vi "DriveForward.vi"(0 "LeftEncoder":T13={"DevStatus"={"status"=FALSE, "code"=0, "source"=""}, "EncoderIndex"=enum."Invalid", "CounterIndex"=enum."Invalid", "DistancePerCount"=1.0, "Decoding Type"=enum."4x"}, 1 "RightEncoder":T13={"DevStatus"={"status"=FALSE, "code"=0, "source"=""}, "EncoderIndex"=enum."Invalid", "CounterIndex"=enum."Invalid", "DistancePerCount"=1.0, "Decoding Type"=enum."4x"}, 2 "Inches to Travel":dbl, 4 "Drive":T3={"DevStatus"={"status"=FALSE, "code"=0, "source"=""}, "Motors[]"=[], "Square Inputs"=FALSE, "Max Output"=1.0}, 5 "Max":dbl, 6 "Transmission":T1={"DevStatus"={"status"=FALSE, "code"=0, "source"=""}, "Pneumatics Control Module"=0, "Forward Solenoid Channel"=enum."Invalid", "Reverse Solenoid Channel"=enum."Invalid"}) -> ()   [LabVIEW 2014]
uses:
  <vilib>/Rock Robotics/WPI/Encoder/WPI_EncoderDevRef.ctl
  <vilib>/Rock Robotics/SystemInterfaces/Encoder/FPGA_EncoderIdx.ctl
  <vilib>/Rock Robotics/SystemInterfaces/Counter/FPGA_CounterCtrSystemIndex.ctl
  <vilib>/Rock Robotics/WPI/Encoder/WPI_EncoderType.ctl
  <vilib>/Rock Robotics/WPI/RobotDrive/WPI_RobotDriveDevRef.ctl
  <vilib>/Rock Robotics/WPI/MotorControl/WPI_MotorControlDeviceRef.ctl
  <vilib>/Rock Robotics/WPI/MotorControl/WPI_MotorControlType.ctl
  <vilib>/Rock Robotics/SystemInterfaces/Typedef/FPGA_TypedefDigitalModule.ctl
  <vilib>/Rock Robotics/SystemInterfaces/DIO/FPGA_DIOPWMChannel.ctl
  <vilib>/Rock Robotics/WPI/PWM/WPI_PWMDeadband.ctl
  <vilib>/Rock Robotics/WPI/CAN/Jaguar/SubVIs/WPI_CANJaguar_ControlMode.ctl
  <vilib>/Rock Robotics/WPI/CAN/TalonSRX/WPI_CANTalonSRX_APIControlMode.ctl
  <vilib>/Rock Robotics/WPI/PWM/WPI_PWMTransform_ConPane.ctl
  <vilib>/Rock Robotics/WPI/Solenoid/WPI_SolenoidDevRef.ctl
  <vilib>/Rock Robotics/WPI/Solenoid/WPI_SolenoidChannel.ctl
  <vilib>/addons/control/pid/pid.llb/PID (DBL).vi
  <vilib>/addons/control/pid/NI_PID_pid.lvlib
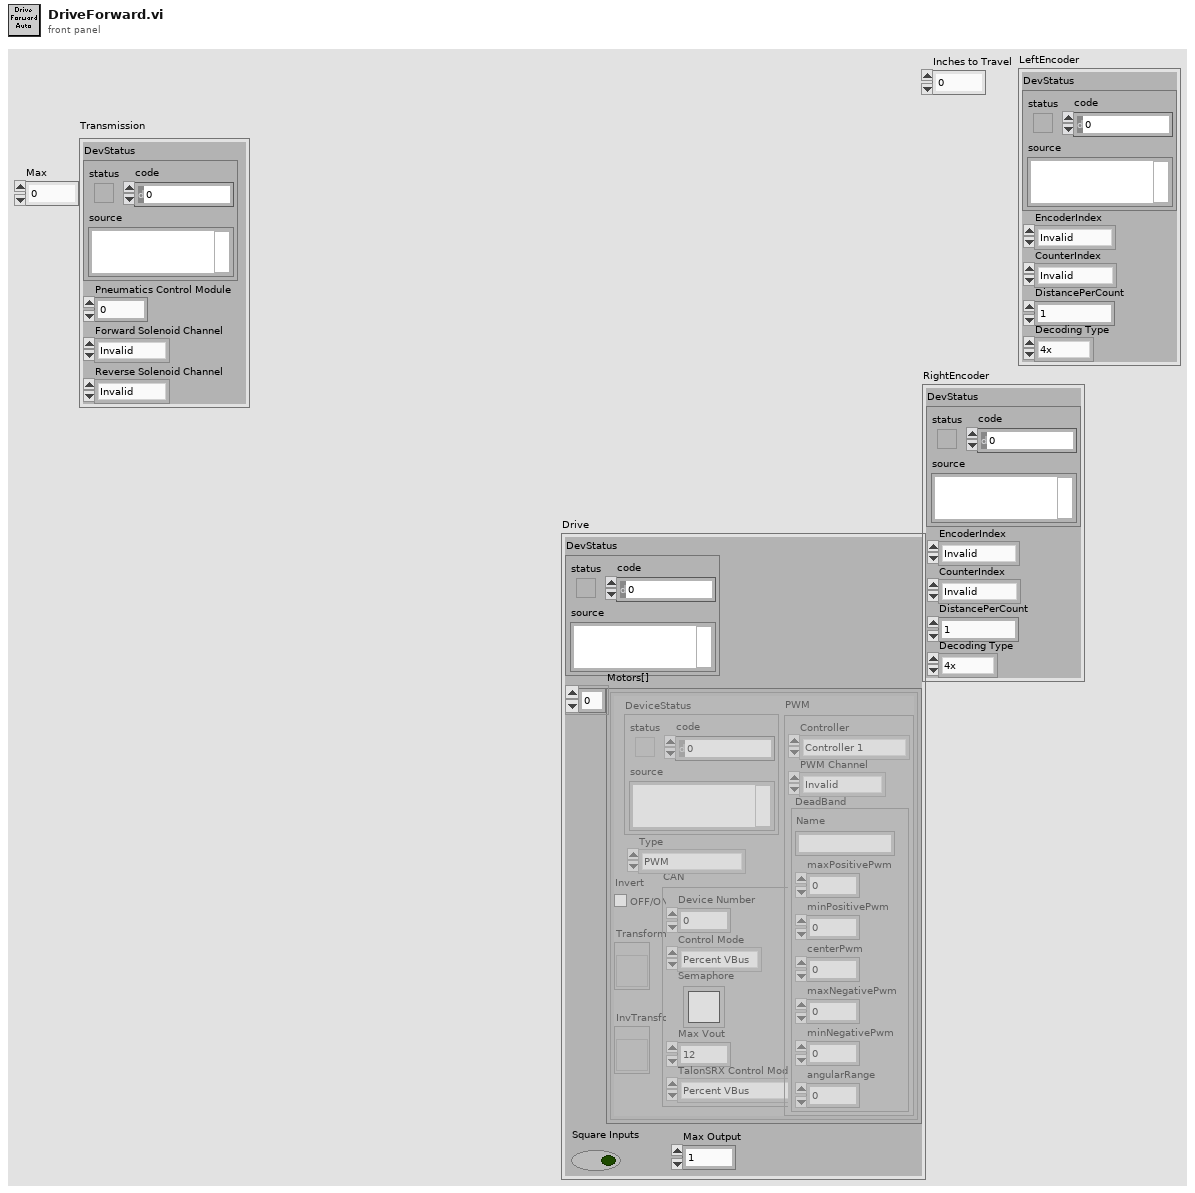
[diagram p1: front panel]
types:
  T1 = typedef "WPI_SolenoidDevRef.ctl" = cluster{"DevStatus":errorcluster, "Pneumatics Control Module":u8, "Forward Solenoid Channel":T2, "Reverse Solenoid Channel":T2}
  T2 = typedef "WPI_SolenoidChannel.ctl" = enum8{"Solenoid 0", "Solenoid 1", "Solenoid 2", "Solenoid 3", "Solenoid 4", "Solenoid 5", "Solenoid 6", "Solenoid 7", "Invalid"}
  T3 = typedef "WPI_RobotDriveDevRef.ctl" = cluster{"DevStatus":errorcluster, "Motors[]":T4[], "Square Inputs":bool, "Max Output":dbl}
  T4 = typedef "WPI_MotorControlDeviceRef.ctl" = cluster{"DeviceStatus":errorcluster, "Type":T5, "PWM":cluster{"Controller":T6, "PWM Channel":T7, "DeadBand":T8}, "CAN":cluster{"Device Number":u8, "Control Mode":T9, "Semaphore":T10, "Max Vout":dbl, "TalonSRX Control Mode":T11}, "Invert":bool, "TransformRef":T12, "InvTransformRef":T12}
  T5 = typedef "WPI_MotorControlType.ctl" = enum16{"PWM", "CAN", "CANTalonSRX"}
  T6 = typedef "FPGA_TypedefDigitalModule.ctl" = enum16{"Controller 1"}
  T7 = typedef "FPGA_DIOPWMChannel.ctl" = enum8{"PWM 0", "PWM 1", "PWM 2", "PWM 3", "PWM 4", "PWM 5", "PWM 6", "PWM 7", "PWM 8", "PWM 9", "PWM MXP 0", "PWM MXP 1", "PWM MXP 2", "PWM MXP 3", "PWM MXP 4", "PWM MXP 5", "PWM MXP 6", "PWM MXP 7", "PWM MXP 8", "PWM MXP 9", "Invalid"}
  T8 = typedef "WPI_PWMDeadband.ctl" = cluster{"Name":string, "maxPositivePwm":i32, "minPositivePwm":i32, "centerPwm":i32, "maxNegativePwm":i32, "minNegativePwm":i32, "angularRange":u16}
  T9 = typedef "WPI_CANJaguar_ControlMode.ctl" = enum8{"Percent VBus", "Current", "Speed", "Position", "Voltage"}
  T10 = typedef "Semaphore RefNum" = refnum<k1>
  T11 = typedef "WPI_CANTalonSRX_APIControlMode.ctl" = enum8{"Percent VBus", "Speed", "Position", "Slave", "Unchanged / Invalid"}
  T12 = typedef "WPI_PWMTransform_ConPane.ctl" = refnum<vi>
  T13 = typedef "WPI_EncoderDevRef.ctl" = cluster{"DevStatus":errorcluster, "EncoderIndex":T14, "CounterIndex":T15, "DistancePerCount":dbl, "Decoding Type":T16}
  T14 = typedef "FPGA_EncoderIdx.ctl" = enum8{"Enc 0", "Enc 1", "Enc 2", "Enc 3", "Enc 4", "Enc 5", "Enc 6", "Enc 7", "Invalid"}
  T15 = typedef "FPGA_CounterCtrSystemIndex.ctl" = enum8{"Ctr 0", "Ctr 1", "Ctr 2", "Ctr 3", "Ctr 4", "Ctr 5", "Ctr 6", "Ctr 7", "Invalid"}
  T16 = typedef "WPI_EncoderType.ctl" = enum16{"1x", "2x", "4x"}
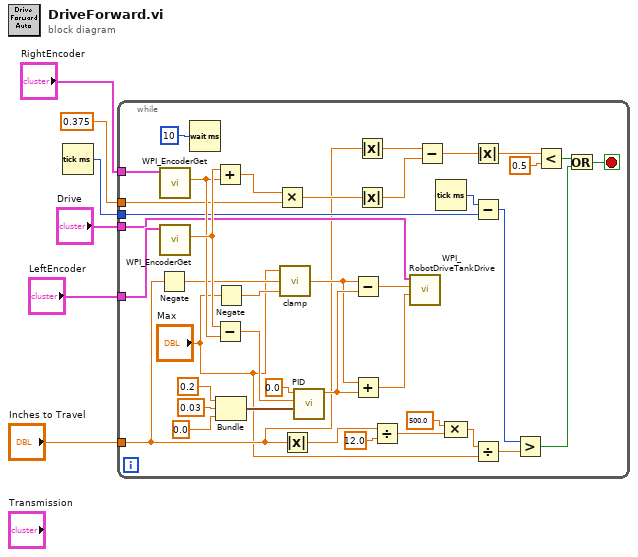
[diagram p0: block diagram]
diagram:
  n1 = Tick Count (ms)() -> (millisecond timer value=w1:u32)
  n2 = while {
    tunnel: "LeftEncoder" -> [w38]
    tunnel: "RightEncoder" -> [w37]
    tunnel: "Drive" -> [w36]
    tunnel: "Inches to Travel" -> [w18]
    tunnel: 0.375 ("t") -> [w28]
    tunnel: w1 -> [w19]
    stop <- w16 stop-if-true
    n3 = Negate(x=w18) -> (-x=w24:dbl)
    n4 = call <vilib>:"WPI_EncoderGet.vi"("EncoderDevRef"=w37) -> ("Distance"=w39:dbl)  [unwired: 5 in, 5 out]
    n5 = call <vilib>:"WPI_EncoderGet.vi"("EncoderDevRef"=w38) -> ("Distance"=w40:dbl)  [unwired: 5 in, 5 out]
    n6 = Wait (ms)(milliseconds to wait=u32 10) -> ()  [unwired: 1 out]
    n7 = Add(x=w40, y=w39) -> (x+y=w29:dbl)
    n8 = Subtract(x=w40, y=w39) -> (x-y=w41:dbl)
    n9 = Negate(x="Max") -> (-x=w30:dbl)
    n10 = Bundle(0.2, 0.03, 0.0) -> (w43:cluster{dbl, dbl, dbl})  [unwired: 1 in]
    n11 = Multiply(x=w29, y=w28) -> (x*y=w22:dbl)
    n12 = call "clamp.vi"("Min"=w30, "Input"=w24, "Max"="Max") -> ("Output"=w31:dbl)
    n13 = Absolute Value(x=w18) -> (abs(x)=w13:dbl)
    n14 = call-poly <vilib>:"PID.vi"("PID gains"=w43, "process variable"=w41, "setpoint"=0.0) -> ("output"=w35:dbl)  [unwired: 7 in, 1 out]
    n15 = Subtract(x=w31, y=w35) -> (x-y=w33:dbl)
    n16 = Add(x=w31, y=w35) -> (x+y=w34:dbl)
    n17 = Absolute Value(x=w18) -> (abs(x)=w23:dbl)
    n18 = Absolute Value(x=w22) -> (abs(x)=w21:dbl)
    n19 = Divide(x=w13, y=12.0) -> (x/y=w11:dbl)
    n20 = call <vilib>:"WPI_RobotDriveTankDrive.vi"("Right axis value"=w34, "Left axis value"=w33, "RobotDriveDevRef"=w36) -> ()  [unwired: 6 in, 3 out]
    n21 = Subtract(x=w23, y=w21) -> (x-y=w27:dbl)
    n22 = Tick Count (ms)() -> (millisecond timer value=w20:u32)
    n23 = Compound Arithmetic op=MULTIPLY(500.0 ("value"), w11) -> (w9:dbl)
    n24 = Absolute Value(x=w27) -> (abs(x)=w26:dbl)
    n25 = Subtract(x=w20, y=w19) -> (x-y=w17:u32)
    n26 = Divide(x=w9, y="Max") -> (x/y=w10:dbl)
    n27 = Greater?(x=w17, y=w10) -> (0:w15:bool)
    n28 = Less?(x=w26, y=0.5) -> (x < y?=w14:bool)
    n29 = Or(x=w14, y=w15) -> (x .or. y?=w16:bool)
  }
